vi "Finish.vi"   [LabVIEW 2018]
doc: "This VI is called just before exiting. It is expected to close I/O refnum, save collected data, etc."
types:
  T1 = typedef "WPI_MotorControlDeviceRef.ctl" = cluster{"DeviceStatus":errorcluster, "Type":T2, "PWM":cluster{"PWM Channel":T3, "DeadBand":T4}, "CAN":cluster{"Device Number":u8, "SetOutput VI Ref":variant, "GetOutput VI Ref":variant, "Enable VI Ref":variant, "Disable VI Ref":variant, "Data":variant}, "Invert":bool, "DIO PWM":cluster{"PWM \"Enable\" Channel":T3, "DIOChannel":T5, "PWM Rate":dbl}}
  T2 = typedef "WPI_MotorControlType.ctl" = enum16{"PWM", "CAN", "DIO PWM"}
  T3 = typedef "FPGA_DIOPWMChannel.ctl" = enum8{"PWM 0", "PWM 1", "PWM 2", "PWM 3", "PWM 4", "PWM 5", "PWM 6", "PWM 7", "PWM 8", "PWM 9", "PWM MXP 0", "PWM MXP 1", "PWM MXP 2", "PWM MXP 3", "PWM MXP 4", "PWM MXP 5", "PWM MXP 6", "PWM MXP 7", "PWM MXP 8", "PWM MXP 9", "Invalid"}
  T4 = typedef "WPI_PWMDeadband.ctl" = cluster{"Name":string, "maxPositivePwm":i32, "minPositivePwm":i32, "centerPwm":i32, "maxNegativePwm":i32, "minNegativePwm":i32, "angularRange":u16}
  T5 = typedef "FPGA_DIOChannel.ctl" = enum8{"DIO 0", "DIO 1", "DIO 2", "DIO 3", "DIO 4", "DIO 5", "DIO 6", "DIO 7", "DIO 8", "DIO 9", "DIO MXP 0", "DIO MXP 1", "DIO MXP 2", "DIO MXP 3", "DIO MXP 4", "DIO MXP 5", "DIO MXP 6", "DIO MXP 7", "DIO MXP 8", "DIO MXP 9", "DIO MXP 10", "DIO MXP 11", "DIO MXP 12", "DIO MXP 13", "DIO MXP 14", "DIO MXP 15", "SPI Port CS1", "SPI Port CS2", "SPI Port CS3", "SPI Port MISO", "SPI Port MOSI", "Invalid"}
  T6 = typedef "WPI_JoystickDevRef.ctl" = cluster{"Device":T7}
  T7 = typedef "WPI_JoystickDeviceEnum.ctl" = enum16{"USB 0", "USB 1", "USB 2", "USB 3", "USB 4", "USB 5"}
  T8 = typedef "WPI_RobotDriveDevRef.ctl" = cluster{"DevStatus":errorcluster, "Motors[]":T1[], "Square Inputs":bool, "Max Output":dbl}
  T9 = typedef "WPI_CompressorDevRef.ctl" = cluster{"DevStatus":errorcluster, "Pneumatics Control Module":u8}
  T10 = typedef "WPI_EncoderDevRef.ctl" = cluster{"DevStatus":errorcluster, "EncoderIndex":T11, "CounterIndex":T12, "DistancePerCount":dbl, "Decoding Type":T13}
  T11 = typedef "FPGA_EncoderIdx.ctl" = enum8{"Enc 0", "Enc 1", "Enc 2", "Enc 3", "Enc 4", "Enc 5", "Enc 6", "Enc 7", "Invalid"}
  T12 = typedef "FPGA_CounterCtrSystemIndex.ctl" = enum8{"Ctr 0", "Ctr 1", "Ctr 2", "Ctr 3", "Ctr 4", "Ctr 5", "Ctr 6", "Ctr 7", "Invalid"}
  T13 = typedef "WPI_EncoderType.ctl" = enum16{"1x", "2x", "4x"}
  T14 = typedef "WPI_GyroDevRef.ctl" = cluster{"DevStatus":errorcluster, "Analog Channel":T15, "Gain (VoltsPerDegree/Second)":dbl, "Gyro Type":enum16{"Analog", "XRS450"}, "Handle":i32, "SPI Bus":T16, "Device Found":bool, "Sample Rate":dbl, "Calibrate On Open":bool, "Offset":dbl}
  T15 = typedef "FPGA_AIChannel.ctl" = enum8{"AI 0", "AI 1", "AI 2", "AI 3", "AI MXP 0", "AI MXP 1", "AI MXP 2", "AI MXP 3", "Invalid"}
  T16 = typedef "spi_bus.ctl" = enum16{"SPI On-Board, CS0", "SPI On-Board, CS1", "SPI On-Board, CS2", "SPI On-Board, CS3", "SPI MXP", "Invalid"}
  T17 = typedef "WPI_AccelerometerDevRef.ctl" = cluster{"DevStatus":errorcluster, "Scaling":T18, "Analog Channels":T19, "I2C Bus":T20, "SPI Bus":T16, "Accel Range":T21, "ADXL Axes":T22, "Handle":i32, "Device Address":u8, "Accel Type":enum16{"Analog", "ADXL345 I2C", "ADXL345 SPI", "Internal", "ADXL362 SPI"}}
  T18 = typedef "WPI_AccelerometerScaling.ctl" = cluster{"Gain (VoltsPerG)":dbl, "Center Voltage":dbl}
  T19 = typedef "WPI_AccelerometerAnalogChannels.ctl" = cluster{"X-Axis":T15, "Y-Axis":T15, "Z-Axis":T15}
  T20 = typedef "i2c_bus.ctl" = enum16{"I2C On-Board", "I2C MXP", "Invalid"}
  T21 = typedef "ADXL345 Range.ctl" = u8
  T22 = typedef "WPI_AccelerometerADXL345 Axes.ctl" = cluster{"X-Axis":bool, "Y-Axis":bool, "Z-Axis":bool}
  T23 = typedef "WPI_AnalogChannelDevRef.ctl" = cluster{"DevStatus":errorcluster, "Analog Channel":T15}
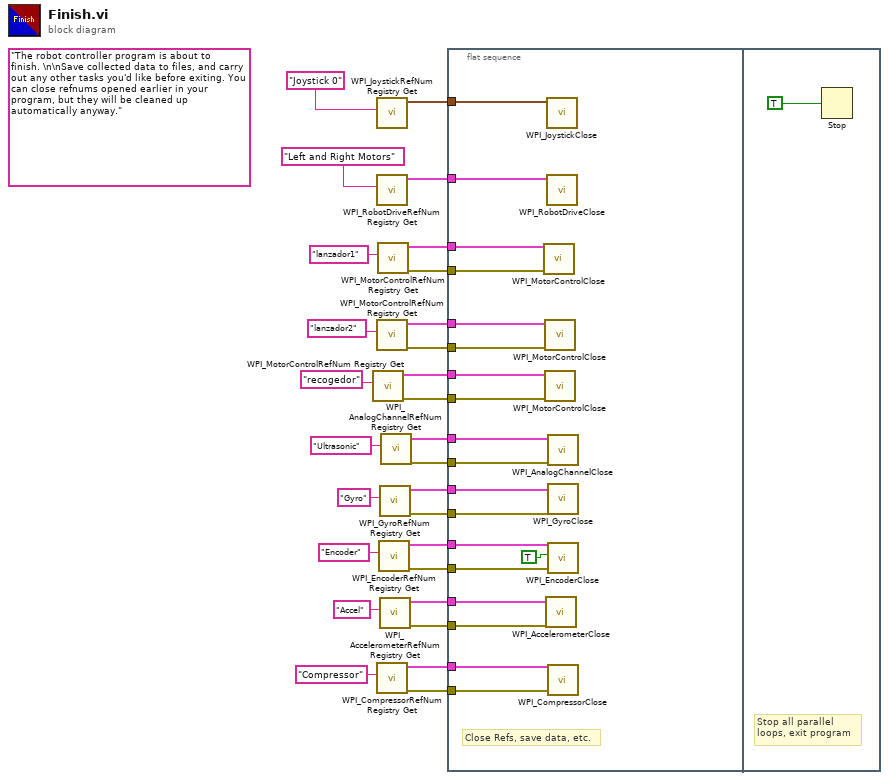
[diagram p0: block diagram]
diagram:
  (unwired) "The robot controller program is about to finish. \n\nSave collected data to files, and carry out any other tasks you'd like before exiting. You can close refnums opened earlier in your program, but they will be cleaned up automatically anyway."
  n1 = call <vilib>:"WPI_MotorControlRefNum Registry Get.vi"("refnum name"="recogedor") -> ("error out"=w16:errorcluster, "MotorControlDevRef"=w17:T1)  [unwired: 9 in]
  n2 = call <vilib>:"WPI_JoystickRefNum Registry Get.vi"("refnum name"="Joystick 0") -> ("JoystickDevRef"=w25:T6)  [unwired: 1 in, 9 out]
  n3 = call <vilib>:"WPI_RobotDriveRefNum Registry Get.vi"("refnum name"="Left and Right Motors") -> ("RobotDriveDevRef"=w26:T8)  [unwired: 1 in, 9 out]
  n4 = call <vilib>:"WPI_MotorControlRefNum Registry Get.vi"("refnum name"="lanzador2") -> ("error out"=w19:errorcluster, "MotorControlDevRef"=w20:T1)  [unwired: 9 in]
  n5 = call <vilib>:"WPI_CompressorRefNum Registry Get.vi"("refnum name"="Compressor") -> ("error out"=w2:errorcluster, "CompressorDevRef"=w3:T9)  [unwired: 9 in]
  n6 = call <vilib>:"WPI_MotorControlRefNum Registry Get.vi"("refnum name"="lanzador1") -> ("error out"=w23:errorcluster, "MotorControlDevRef"=w24:T1)  [unwired: 9 in]
  n7 = call <vilib>:"WPI_EncoderRefNum Registry Get.vi"("refnum name"="Encoder") -> ("error out"=w8:errorcluster, "EncoderDevRef"=w9:T10)  [unwired: 9 in]
  n8 = call <vilib>:"WPI_GyroRefNum Registry Get.vi"("refnum name"="Gyro") -> ("error out"=w11:errorcluster, "GyroDevRef"=w12:T14)  [unwired: 9 in]
  n9 = call <vilib>:"WPI_AccelerometerRefNum Registry Get.vi"("refnum name"="Accel") -> ("error out"=w5:errorcluster, "AccelerometerDevRef"=w6:T17)  [unwired: 9 in]
  n10 = call <vilib>:"WPI_AnalogChannelRefNum Registry Get.vi"("refnum name"="Ultrasonic") -> ("error out"=w14:errorcluster, "AIDeviceRef"=w15:T23)  [unwired: 9 in]
  n11 = flat-sequence {
    tunnel: w26 -> [w47]
    tunnel: w25 -> [w46]
    tunnel: w24 -> [w45]
    tunnel: w23 -> [w44]
    tunnel: w20 -> [w43]
    tunnel: w19 -> [w42]
    tunnel: w17 -> [w41]
    tunnel: w16 -> [w40]
    tunnel: w15 -> [w39]
    tunnel: w14 -> [w38]
    tunnel: w12 -> [w37]
    tunnel: w11 -> [w36]
    tunnel: w9 -> [w35]
    tunnel: w8 -> [w34]
    tunnel: w6 -> [w32]
    tunnel: w5 -> [w31]
    tunnel: w3 -> [w30]
    tunnel: w2 -> [w29]
    frame #0 {
      # "Close Refs, save data, etc."
      n12 = call <vilib>:"WPI_MotorControlClose.vi"("error in"=w44, "MotorControlDevRef"=w45) -> ()  [unwired: 9 in, 1 out]
      n13 = call <vilib>:"WPI_MotorControlClose.vi"("error in"=w42, "MotorControlDevRef"=w43) -> ()  [unwired: 9 in, 1 out]
      n14 = call <vilib>:"WPI_MotorControlClose.vi"("error in"=w40, "MotorControlDevRef"=w41) -> ()  [unwired: 9 in, 1 out]
      n15 = call <vilib>:"WPI_AccelerometerClose.vi"("error in"=w31, "AccelerometerDevRef"=w32) -> ()  [unwired: 9 in, 1 out]
      n16 = call <vilib>:"WPI_JoystickClose.vi"("JoystickDevRef"=w46) -> ()  [unwired: 11 out]
      n17 = call <vilib>:"WPI_RobotDriveClose.vi"("RobotDriveDevRef"=w47) -> ()  [unwired: 1 in, 10 out]
      n18 = call <vilib>:"WPI_AnalogChannelClose.vi"("error in (no error)"=w38, "AIDeviceRef"=w39) -> ()  [unwired: 9 in, 1 out]
      n19 = call <vilib>:"WPI_GyroClose.vi"("error in"=w36, "GyroDevRef"=w37) -> ()  [unwired: 9 in, 1 out]
      n20 = call <vilib>:"WPI_EncoderClose.vi"("error in (no error)"=w34, "Close Dependencies"=TRUE, "EncoderDevRef"=w35) -> ()  [unwired: 8 in, 1 out]
      n21 = call <vilib>:"WPI_CompressorClose.vi"("error in (no error)"=w29, "CompressorDevRef"=w30) -> ()  [unwired: 9 in, 1 out]
    }
    frame #1 {
      # "Stop all parallel\nloops, exit program"
      n22 = Stop(stop? (T)=TRUE ("Quit")) -> ()
    }
  }
